vi "Standart Sapma.vi"() -> ()   [LabVIEW 2015]
uses:
  <vilib>/Utility/file.llb/Read Delimited Spreadsheet (DBL).vi
  <vilib>/Analysis/NI_AALBase.lvlib
panel:
  out "Veriler":dbl[][](array[numeric])
  in  "Okunacak Veri Adresi":path
  out "Standart Sapma":dbl
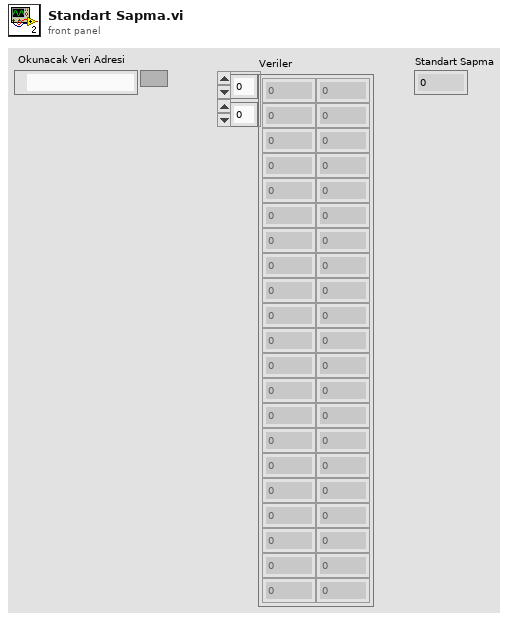
[diagram p1: front panel]
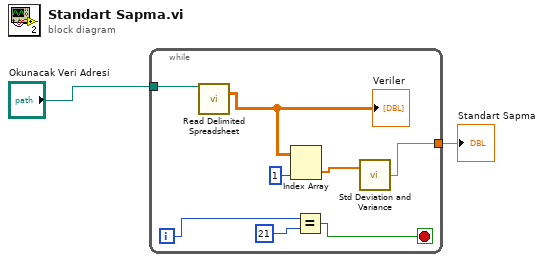
[diagram p0: block diagram]
diagram:
  n1 = while {
    tunnel: "Okunacak Veri Adresi" -> [w10]
    tunnel: [w3] -> w1
    i -> [w8]
    stop <- w6 stop-if-true
    n2 = call-poly <vilib>:"Read Delimited Spreadsheet.vi"("file path (dialog if empty)"=w10) -> ("all rows"=w9:dbl[][])  [unwired: 9 in, 5 out]
    "Veriler" <- w9
    n3 = Index Array(array=w9, index (col)=1 ("disabled index (col)")) -> (element=w4:dbl[])  [unwired: 1 in]
    n4 = Equal?(x=w8, y=21) -> (x = y?=w6:bool)
    n5 = call <vilib>:"Std Deviation and Variance.vi"("X"=w4) -> ("standard deviation"=w3:dbl)  [unwired: 1 in, 2 out]
  }
  "Standart Sapma" <- w1
